vi "Update Feedback.vi"(6 "Time":dbl, 8 "error in (no error)":errorcluster, 11 "2WayValve in":refnum<class "2WayValve.lvclass">) -> (0 "error out":errorcluster, 3 "2WayValve out":refnum<class "2WayValve.lvclass">)   [LabVIEW 2020, in "VolatusGUI.lvlib" / "2WayValve.lvclass"]
uses:
  2WayValve.lvclass
  2WayValve.lvclass/2WayValve.ctl
  lv-vecto/Vecto/Channel/Channel.lvclass
  lv-vecto/Vecto/Vecto.lvlib
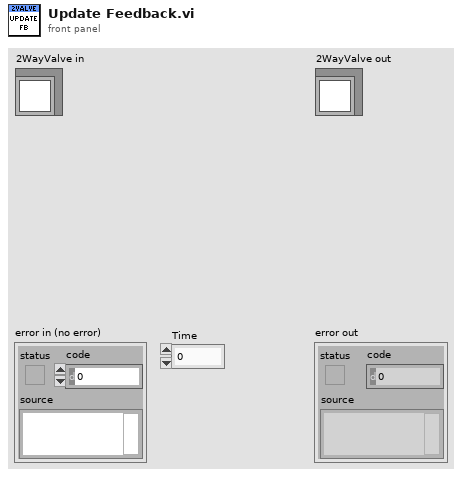
[diagram p1: front panel]
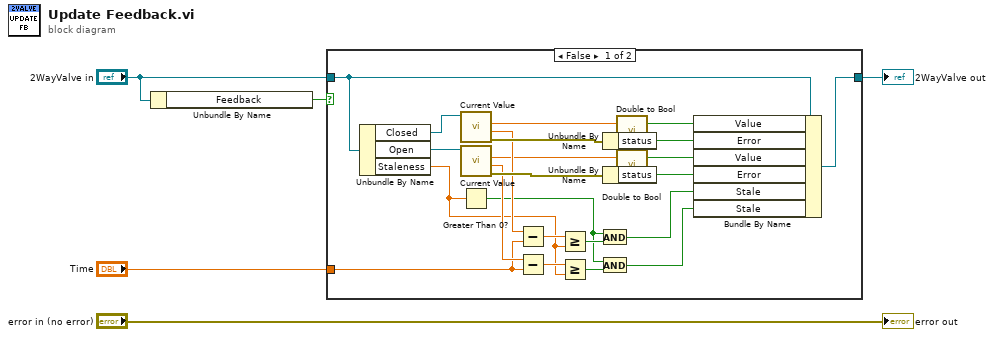
[diagram p0: block diagram]
diagram:
  n1 = Unbundle By Name("2WayValve in") -> ("Feedback"=w4:bool)
  n2 = case shown="False" w4 {
    tunnel: "2WayValve in" -> [w16 w29]
    tunnel: [w6 w29] -> w2
    tunnel: "Time" -> [w22 _]
    frame False {
      n3 = Unbundle By Name(w16) -> ("Closed"=w26:refnum<class "Channel.lvclass">, "Open"=w25:refnum<class "Channel.lvclass">, "Staleness"=w19:dbl)
      n4 = call "Current Value.vi"("Channel in"=w26) -> ("error out"=w28:errorcluster, "Timestamp"=w23:dbl, "Scaled"=w18:dbl)  [unwired: 6 in, 2 out]
      n5 = call "Current Value.vi"("Channel in"=w25) -> ("error out"=w27:errorcluster, "Timestamp"=w24:dbl, "Scaled"=w17:dbl)  [unwired: 6 in, 2 out]
      n6 = Greater Than 0?(x=w19) -> (x > 0?=w9:bool)
      n7 = Subtract(x=w23, y=w22) -> (x-y=w21:dbl)
      n8 = Subtract(x=w24, y=w22) -> (x-y=w20:dbl)
      n9 = Greater Or Equal?(x=w21, y=w19) -> (x >= y?=w11:bool)
      n10 = Greater Or Equal?(x=w20, y=w19) -> (x >= y?=w10:bool)
      n11 = And(x=w9, y=w11) -> (x .and. y?=w8:bool)
      n12 = And(x=w9, y=w10) -> (x .and. y?=w7:bool)
      n13 = Unbundle By Name(w28) -> ("status"=w14:bool)
      n14 = Unbundle By Name(w27) -> ("status"=w12:bool)
      n15 = call "Double to Bool.vi"("Double"=w18) -> ("Bool"=w15:bool)  [unwired: 2 in]
      n16 = call "Double to Bool.vi"("Double"=w17) -> ("Bool"=w13:bool)  [unwired: 2 in]
      n17 = Bundle By Name(cluster=w16, "Value"=w15, "Error"=w14, "Value"=w13, "Error"=w12, "Stale"=w8, "Stale"=w7) -> (w6:refnum<class "2WayValve.lvclass">)
    }
    frame True {
      # "Feedback unused"
    }
  }
  "2WayValve out" <- w2
  "error out" <- "error in (no error)"
